vi "exercise3.vi"() -> ()   [LabVIEW 2010]
panel:
  out "Remainder":dbl
  out "Quotient":dbl
  out "Divide by Zero":bool
  out "Random Number":dbl format="%.7f"
  in  "Divide Result":dbl
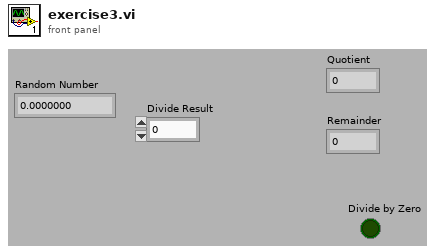
[diagram p1: front panel]
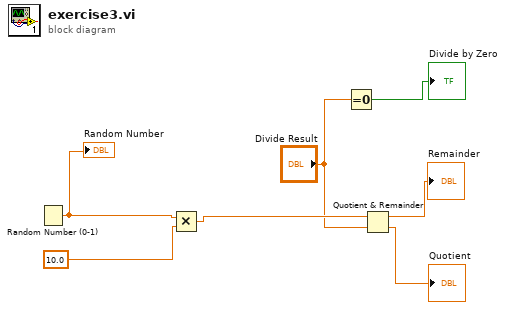
[diagram p0: block diagram]
diagram:
  n1 = Random Number (0-1)() -> (number: 0 to 1=w7:dbl)
  "Random Number" <- w7
  n2 = Multiply(x=w7, y=10.0) -> (x*y=w2:dbl)
  n3 = Equal To 0?(x="Divide Result") -> (x = 0?=→"Divide by Zero":bool)
  n4 = Quotient & Remainder(x=w2, y="Divide Result") -> (x-y*floor(x/y)=→"Remainder":dbl, floor(x/y)=→"Quotient":dbl)
